vi "ReadTemp.vi"(8 "error in (no error)":errorcluster, 10 "Port Number":u16=2000, 11 "IP Address":string="192.168.12.200") -> (0 "error out":errorcluster, 3 "Temperature":dbl format="%.2f")   [LabVIEW 2013, in "ovenCtrl.lvlib"]
uses:
  ovenCtrl.lvlib
panel:
  # "Inputs"
  # "Outputs"
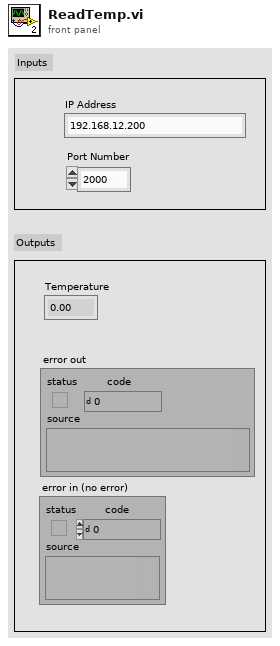
[diagram p1: front panel]
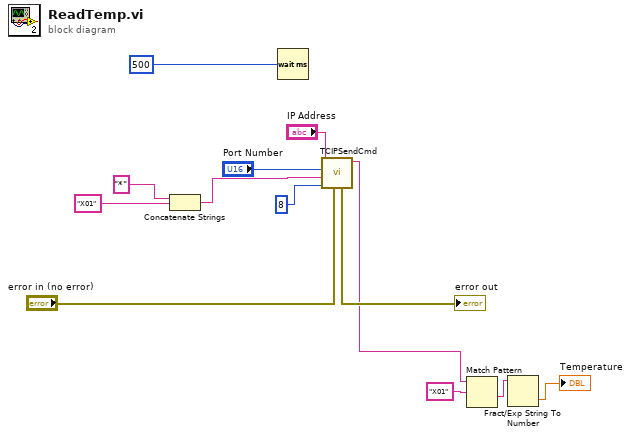
[diagram p0: block diagram]
diagram:
  n1 = Concatenate Strings("*" ("string"), "X01" ("string")) -> (w8:string)
  n2 = Wait (ms)(milliseconds to wait=u32 500) -> ()  [unwired: 1 out]
  n3 = call "TCIPSendCmd.vi"("error in (no error)"="error in (no error)", "bytes to read"=8, "Command"=w8, "Port Number"="Port Number", "IP Address"="IP Address") -> ("Output Reading"=w3:string, "error out"=→"error out":errorcluster)  [unwired: 5 in]
  n4 = Match Pattern(string=w3, regular expression="X01") -> (after substring=w2:string)  [unwired: 1 in, 3 out]
  n5 = Fract/Exp String To Number(string=w2) -> (number=→"Temperature":dbl)  [unwired: 3 in, 1 out]
